vi "Write and Read Multiple Holding Registers.vi"(4 "read count":u16, 6 "read starting address":u16, 8 "error in":errorcluster, 9 "write values":u16[](array[numeric]), 10 "write starting address":u16, 11 "Modbus instance in":refnum<class "Modbus Master.lvclass">) -> (0 "error out":errorcluster, 1 "read values":u16[](array[numeric]), 3 "Modbus instance out":refnum<class "Modbus Master.lvclass">)   [LabVIEW 2015, in "Modbus Library.lvlib" / "Modbus Master.lvclass"]
doc: "Writes and reads the values of multiple register values in series. The <b>write values</b> are inserted starting at <b>write starting address</b> and the returned <b>read values</b> consists of <b>read count</b> holding registers starting at <b>read starting address</b>."
uses:
  Modbus Master.lvclass
  Modbus Master.lvclass/Modbus Master.ctl
  Modbus API.lvclass/Modbus API.ctl
  Transmission Data Unit/Transmission Data Unit.lvclass
  Master Function Definition/Master Function Definition.lvclass
  Modbus API.lvclass
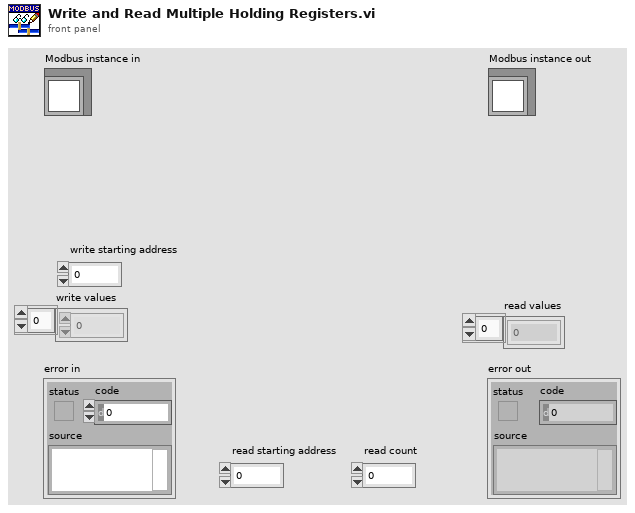
[diagram p1: front panel]
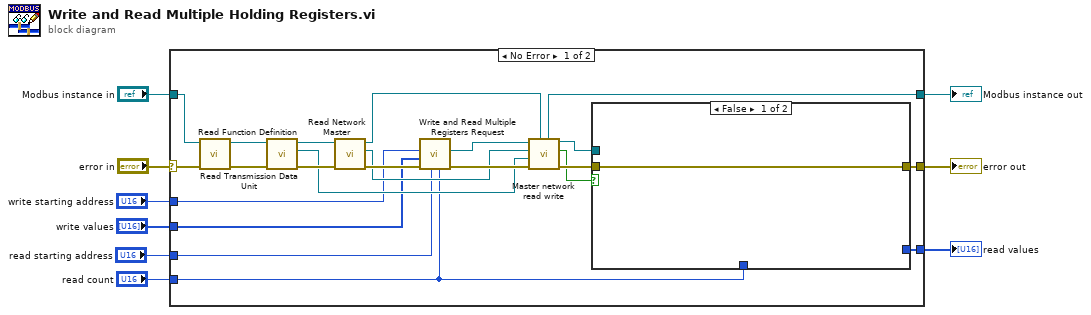
[diagram p0: block diagram]
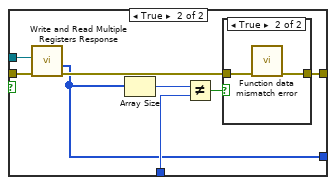
[diagram p2: hidden frame]
diagram:
  n1 = case shown="No Error" "error in" {
    selector: "error in" -> [w21 w44]
    tunnel: "Modbus instance in" -> [w19 w45]
    tunnel: [w26 w45] -> w8
    tunnel: [w30 w44] -> w7
    tunnel: "read count" -> [w15 _]
    tunnel: [w14 _] -> w4
    tunnel: "read starting address" -> [w13 _]
    tunnel: "write values" -> [w12 _]
    tunnel: "write starting address" -> [w11 _]
    frame No Error {
      n2 = call "Read Function Definition.vi"("error in"=w21, "Modbus master in"=w19) -> ("error out"=w24:errorcluster, "Modbus master out"=w23:refnum<class "Modbus Master.lvclass">)  [unwired: 7 in, 1 out]
      n3 = call "Read Transmission Data Unit.vi"("error in"=w24, "Modbus instance in"=w23) -> ("error out"=w22:errorcluster, "transmission data unit"=w17:refnum<class "Transmission Data Unit.lvclass">, "Modbus instance out"=w25:refnum<class "Modbus Master.lvclass">)  [unwired: 7 in]
      n4 = call "Read Network Master.vi"("error in"=w22, "Modbus master in"=w25) -> ("error out"=w20:errorcluster, "network master"=w16:refnum<class "Network Master.lvclass">, "Modbus master out"=w18:refnum<class "Modbus Master.lvclass">)  [unwired: 7 in]
      n5 = call "Write and Read Multiple Registers Request.vi"("Quantity to Read"=w15, "Read Starting Address"=w13, "error in"=w20, "Write"=w12, "Write Starting Address"=w11) -> ("error out"=w31:errorcluster, "modbus data unit out"=w28:refnum<class "Modbus Data Unit.lvclass">)  [unwired: 5 in]
      n6 = call "Master network read write.vi"("Modbus master in"=w18, "error in"=w31, "transmission data unit in"=w17, "network master in"=w16, "Modbus data unit in"=w28) -> ("error out"=w29:errorcluster, "PDU Valid?"=w10:bool, "Modbus data unit out"=w27:refnum<class "Modbus Data Unit.lvclass">, "Modbus master out"=w26:refnum<class "Modbus Master.lvclass">)  [unwired: 3 in]
      n7 = case shown="False" w10 {
        tunnel: [w32 w40] -> w30
        tunnel: w29 -> [w32 w39]
        tunnel: w27 -> [_ w38]
        tunnel: w15 -> [_ w34]
        tunnel: [_ w33] -> w14
        frame False {
        }
        frame True {
          n8 = call "Write and Read Multiple Registers Response.vi"("error in"=w39, "modbus data unit in"=w38) -> ("error out"=w37:errorcluster, "Registers"=w33:u16[])  [unwired: 7 in, 1 out]
          n9 = Array Size(array=w33) -> (size(s)=w35:i32)
          n10 = Not Equal?(x=w35, y=w34) -> (x != y?=w36:bool)
          n11 = case shown="True" w36 {
            tunnel: [w41 w43] -> w40
            tunnel: w37 -> [w41 w42]
            frame False {
            }
            frame True {
              n12 = call "Function data mismatch error.vi"("error in (no error)"=w42) -> ("error out"=w43:errorcluster)  [unwired: 10 in]
            }
          }
        }
      }
    }
    frame Error {
    }
  }
  "error out" <- w7
  "Modbus instance out" <- w8
  "read values" <- w4
